vi "Read Settings from File.vi"(8 "error in (no error)":errorcluster, 11 "Ini path":path) -> (0 "error out":errorcluster, 2 "Store Settings":T1, 3 "Ini out":T2)   [LabVIEW 2015, in "VI App Store.lvlib" / "VIStore.lvclass"]
uses:
  VIStore.lvclass
  <vilib>/Utility/config.llb/Config Data RefNum.ctl
  Classes/Settings Item/Settings Data.ctl
  <vilib>/Utility/config.llb/Read Key (Path).vi
  <vilib>/Utility/config.llb/Read Key (Boolean).vi
  <vilib>/Utility/config.llb/NI_LVConfig.lvlib
  Classes/Settings Item/Settings.lvclass
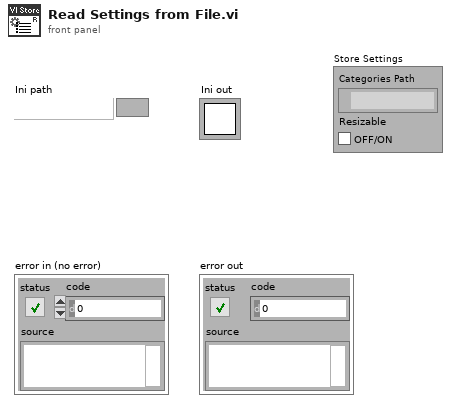
[diagram p1: front panel]
types:
  T1 = typedef "Item Actor.lvlib/Settings.lvclass/Settings Data.ctl" = cluster{"Categories Path":path, "Resizable":bool}
  T2 = typedef "NI_LVConfig.lvlib/Config Data RefNum.ctl" = refnum<k1>
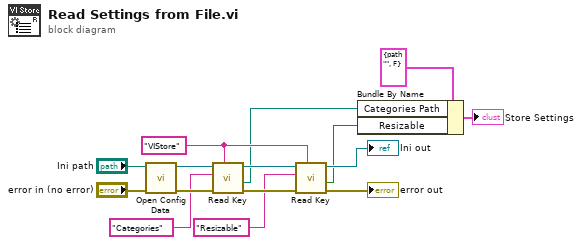
[diagram p0: block diagram]
diagram:
  w9 = "VIStore" ("section")
  n1 = call <vilib>:"Open Config Data.vi"("error in (no error)"="error in (no error)", "configuration file path"="Ini path") -> ("error out"=w12:errorcluster, "refnum"=w6:T2)  [unwired: 7 in, 1 out]
  n2 = call-poly <vilib>:"Read Key.vi"("section"=w9, "error in (no error)"=w12, "key"="Categories", "refnum"=w6) -> ("error out"=w13:errorcluster, "value"=w3:path, "refnum out"=w7:T2)  [unwired: 4 in, 1 out]
  n3 = call-poly <vilib>:"Read Key.vi"("section"=w9, "error in (no error)"=w13, "key"="Resizable", "refnum"=w7) -> ("error out"=→"error out":errorcluster, "value"=w2:bool, "refnum out"=→"Ini out":T2)  [unwired: 4 in, 1 out]
  n4 = Bundle By Name(cluster=T1 {"Categories Path"=path "", "Resizable"=FALSE} ("Settings Data"), "Categories Path"=w3, "Resizable"=w2) -> (→"Store Settings":T1)
